vi "Build Express Waveform.vi"   [LabVIEW 2020]
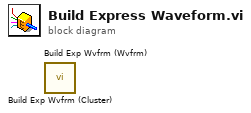
[diagram p0: block diagram]
diagram:
  n1 = call <vilib>:"Build Exp Wvfrm (Wvfrm).vi"() -> ()  [unwired: 10 in, 2 out]
  n2 = call <vilib>:"Build Exp Wvfrm (Cluster).vi"() -> ()  [unwired: 10 in, 2 out]
